vi "LWXPS_SetJogAcceleration.vi"(5 "LabVIEW error IN":errorcluster, 6 "XPS Reference IN":refnum<k24>, 7 "Y Smooth factor":i32, 8 "Y acceleration time":i32, 9 "X Smooth factor":i32, 10 "X acceleration time":i32) -> (0 "LabVIEW error OUT":errorcluster, 1 "XPS Error String":string, 2 "Returned error code":i32, 3 "XPS Reference OUT":refnum<k24>)   [LabVIEW 2014]
uses:
  D:/XPSQ8_LabView_Library/Development/Source/Dll/Newport.XPS.CommandInterface.dll
  Dll/Newport.XPS.CommandInterface.dll
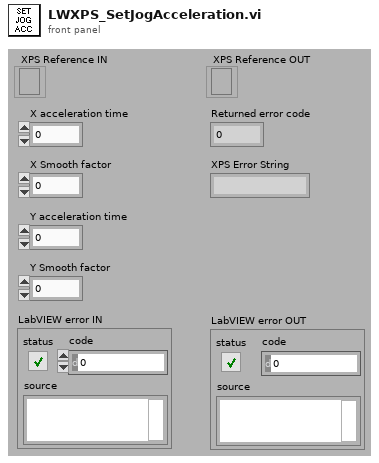
[diagram p1: front panel]
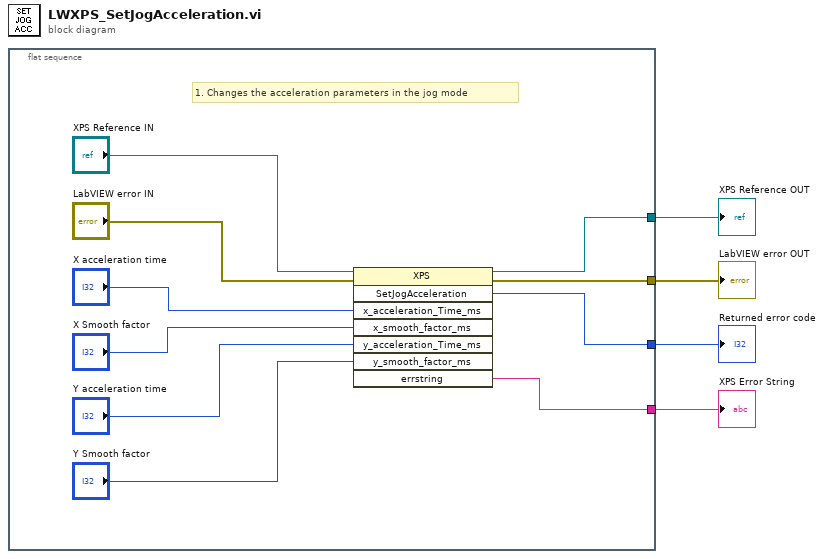
[diagram p0: block diagram]
diagram:
  n1 = flat-sequence {
    tunnel: [w11] -> w4
    tunnel: [w10] -> w3
    tunnel: [w12] -> w2
    tunnel: [w9] -> w1
    frame #0 {
      # "1. Changes the acceleration parameters in the jog mode"
      n2 = invoke class="XPS" method="SetJogAcceleration"(reference="XPS Reference IN", error in="LabVIEW error IN", "x_acceleration_Time_ms"="X acceleration time", "x_smooth_factor_ms"="X Smooth factor", "y_acceleration_Time_ms"="Y acceleration time", "y_smooth_factor_ms"="Y Smooth factor") -> (reference out=w11:refnum<k24>, error out=w10:errorcluster, "SetJogAcceleration"=w12:i32, "errstring"=w9:string)  [unwired: 2 in, 4 out]
    }
  }
  "XPS Error String" <- w1
  "XPS Reference OUT" <- w4
  "LabVIEW error OUT" <- w3
  "Returned error code" <- w2
